vi "log_error.vi"(6 "timestamp":timestamp, 7 "context":string, 8 "error in (no error)":errorcluster, 9 "level":T1=200 items=["OFF"=0, "FATAL"=100, "ERROR"=200, "WARN"=300, "INFO"=400, "DEBUG"=500, "TRACE"=600, "ALL"=65535], 11 "File Log Provider in":refnum<class "File Log Provider.lvclass">) -> (0 "error out":errorcluster, 3 "File Log Provider out":refnum<class "File Log Provider.lvclass">)   [LabVIEW 2019, in "File Log Provider.lvclass"]
uses:
  File Log Provider.lvclass
  Queue Log Provider/Queue Log Provider.lvclass
  Log Service/public/level.ctl
  Log Service/Log Service.lvclass
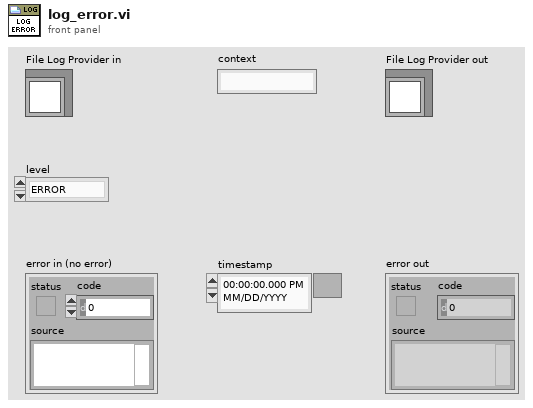
[diagram p1: front panel]
types:
  T1 = typedef "Utility API.lvlib/Log Service.lvclass/level.ctl" = u16
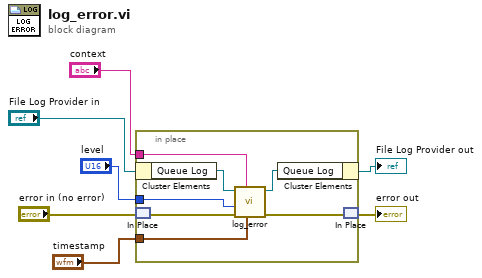
[diagram p0: block diagram]
diagram:
  n1 = in-place {
    in-place-border: "context" -> [w10]
    in-place-border: "level" -> [w9]
    in-place-border: "timestamp" -> [w8]
    n2 = in-place-cluster #1("File Log Provider in") -> ("Queue Log"=w14:refnum<class "Queue Log Provider.lvclass">)
    n3 = in-place-match #2("error in (no error)") -> (w12:errorcluster)
    n4 = call-dynamic "log_error.vi"("timestamp"=w8, "context"=w10, "error in (no error)"=w12, "level"=w9, "Queue Log Provider in"=w14) -> ("error out"=w11:errorcluster, "Queue Log Provider out"=w13:refnum<class "Queue Log Provider.lvclass">)  [unwired: 5 in]
    n5 = in-place-cluster #1("Queue Log"=w13) -> (→"File Log Provider out":refnum<class "File Log Provider.lvclass">)
    n6 = in-place-match #2(w11) -> (→"error out":errorcluster)
  }
